vi "SPOL_temps_PB.vi"() -> ()   [LabVIEW 2009]
uses:
  <vilib>/Utility/file.llb/Read From Spreadsheet File (string).vi
panel:
  out "output array":dbl[](array[numeric])
  in  "Reset\nDisplay":bool
  in  "stop":bool
  in  "Select":bool
  in  "Plot":bool
  in  "History Data":T1(array[cluster])
  out "Labels":string[](array[string])
  out "Housekeeping File":path caption="selected path"
  out "Temperatures":T2(graph)
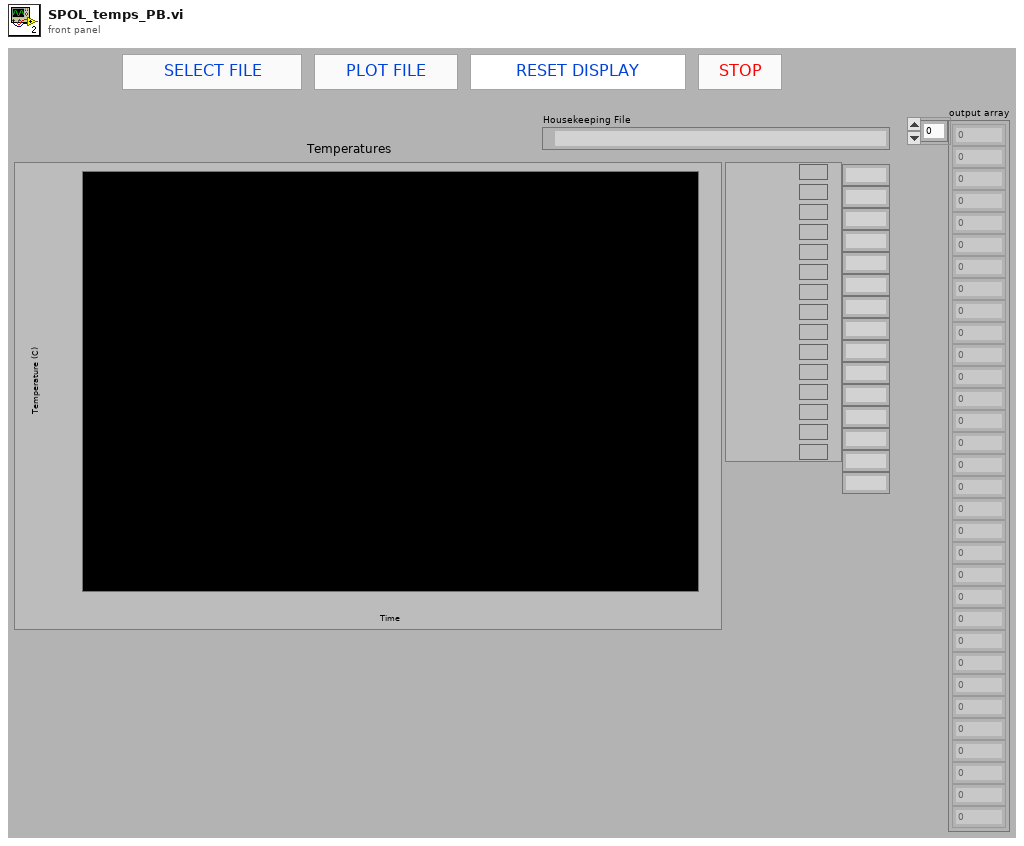
[diagram p1: front panel]
types:
  T1 = cluster{"[0]":dbl, "[1]":dbl, "[2]":dbl, "[3]":dbl, "[4]":dbl, "[5]":dbl, "[6]":dbl, "[7]":dbl, "[8]":dbl, "[9]":dbl, "[10]":dbl, "[11]":dbl, "[12]":dbl, "[13]":dbl, "[14]":dbl}[]
  T2 = cluster{"[0]":dbl, "[1]":dbl, "[2]":dbl, "[3]":dbl, "[4]":dbl, "[5]":dbl, "[6]":dbl, "[7]":dbl, "[8]":dbl, "[9]":dbl, "[10]":dbl, "[11]":dbl, "[12]":dbl, "[13]":dbl, "[14]":dbl}
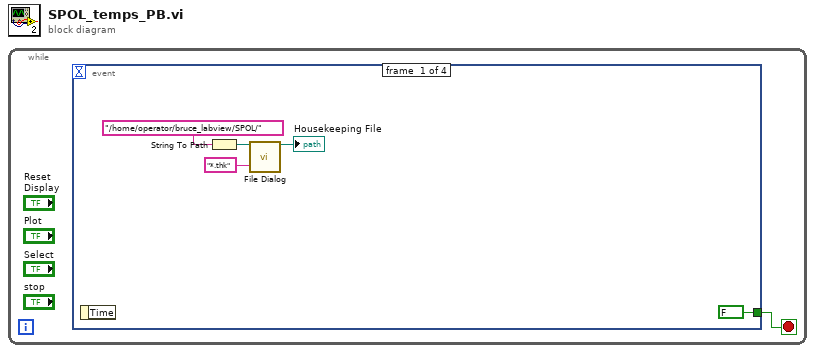
[diagram p0: block diagram]
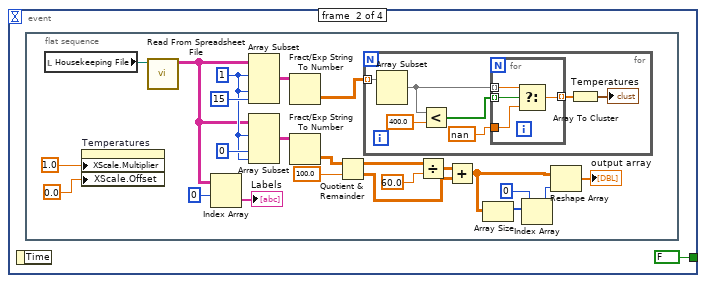
[diagram p2: hidden frame]
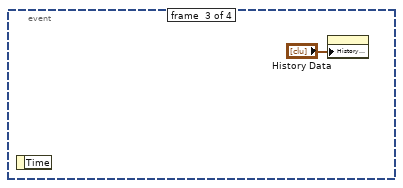
[diagram p3: hidden frame]
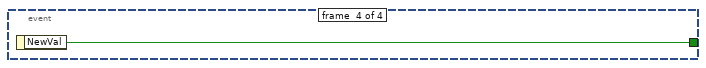
[diagram p4: hidden frame]
diagram:
  n1 = while {
    stop <- w1 stop-if-true
    n2 = event shown="[1] \"Plot\": Value Change" {
      selector: _ -> [_ _ _ _]
      dyn-events: _ -> [_ _ _ _]
      timeout: _ -> [_ _ _ _]
      tunnel: [FALSE ("NewVal") FALSE _ w43] -> w1
      event #0 {
        n3 = event-data() -> ()  [unwired: 1 in, 1 out]
        n4 = String To Path(string="/home/operator/bruce_labview/SPOL/") -> (path=w4:path)
        n5 = call "File Dialog"("start path"=w4, "pattern (all files)"="*.thk") -> ("selected path"=→"Housekeeping File":path)  [unwired: 10 in, 3 out]
      }
      event #1 {
        n6 = event-data() -> ()  [unwired: 1 in, 1 out]
        n7 = flat-sequence {
          frame #0 {
            w25 = 1 ("index")
            n8 = local read "Housekeeping File"() -> (w30:path)
            n9 = property on="Temperatures" class="WFChart (strict)"("XScale.Multiplier"=1.0 ("X Scale.Offset and Multiplier:Multiplier"), "XScale.Offset"=0.0 ("X Scale.Offset and Multiplier:Offset")) -> ()  [unwired: 2 in, 2 out]
            n10 = call-poly <vilib>:"Read From Spreadsheet File.vi"("file path (dialog if empty)"=w30) -> ("all rows"=w22:string[][])  [unwired: 6 in, 4 out]
            n11 = Index Array(array=w22, index (row)=0) -> (element=→"Labels":string[])  [unwired: 1 in]
            n12 = Array Subset(array=w22, index (row)=w25, index (col)=w25, length (col)=15 ("length")) -> (w29:string[][])  [unwired: 1 in]
            n13 = Array Subset(array=w22, index (row)=w25, index (col)=0 ("index"), length (col)=w25) -> (w15:string[][])  [unwired: 1 in]
            n14 = Fract/Exp String To Number(string=w29) -> (number=w27:dbl[][])  [unwired: 3 in, 1 out]
            n15 = Fract/Exp String To Number(string=w15) -> (number=w21:dbl[][])  [unwired: 3 in, 1 out]
            n16 = Quotient & Remainder(x=w21, y=100.0) -> (x-y*floor(x/y)=w19:dbl[][], floor(x/y)=w16:dbl[][])
            n17 = for {
              tunnel: w27 -> [w37] mode=indexing
              n18 = Array Subset(array=w37) -> (w32:dbl[])  [unwired: 2 in]
              n19 = Less?(x=w32, y=400.0 ("element")) -> (x < y?=w31:bool[])
              n20 = for {
                tunnel: w31 -> [w41] mode=indexing
                tunnel: w32 -> [w39] mode=indexing
                tunnel: nan ("number/path/refnum") -> [w40]
                tunnel: [w38] -> w34 mode=indexing
                n21 = Select(t=w39, s=w41, f=w40) -> (s? t:f=w38:dbl)
              }
              n22 = Array To Cluster(array=w34) -> (cluster=→"Temperatures":T2)
            }
            n23 = Divide(x=w19, y=60.0) -> (x/y=w17:dbl[][])
            n24 = Add(x=w17, y=w16) -> (x+y=w12:dbl[][])
            n25 = Array Size(array=w12) -> (size(s)=w11:i32[])
            n26 = Index Array(array=w11, index=0) -> (element=w9:i32)
            n27 = Reshape Array(w12, w9) -> (→"output array":dbl[])
          }
        }
      }
      event #2 {
        n28 = event-data() -> ()  [unwired: 1 in, 1 out]
        n29 = property on="Temperatures" class="WFChart (strict)"("History Data"="History Data") -> ()  [unwired: 2 in, 2 out]
      }
      event #3 {
        n30 = event-data() -> ("NewVal"=w43:bool)  [unwired: 1 in]
      }
    }
  }
